vi "Create Grid.vi"(9 "Height":i32, 10 "Width":i32, 11 "Bounding Coordinates":T3={"Top Left Coordinate"={"Coordinate"=-3.0+1.5i, "Iteration"=0.0, "Escaped? "=FALSE, "Iteration Value"=0.0+0.0i}, "Bottom Right Coordinate"={"Coordinate"=1.0-1.5i, "Iteration"=0.0, "Escaped? "=FALSE, "Iteration Value"=0.0+0.0i}}) -> (3 "Grid":T1[][](array[typedef]))   [LabVIEW 2016]
uses:
  MandelPoint.ctl
panel:
  in  "MandelPointn Dummy":T1
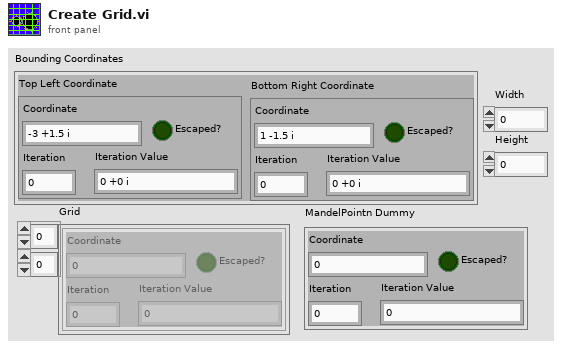
[diagram p1: front panel]
types:
  T1 = typedef "MandelPoint.ctl" = cluster{"Coordinate":cdb, "Iteration":u16, "Escaped? ":bool, "Iteration Value":cdb}
  T2 = typedef "MandelPoint.ctl" = cluster{"Coordinate":cdb, "Iteration":dbl, "Escaped? ":bool, "Iteration Value":cdb}
  T3 = cluster{"Top Left Coordinate":T2, "Bottom Right Coordinate":T2}
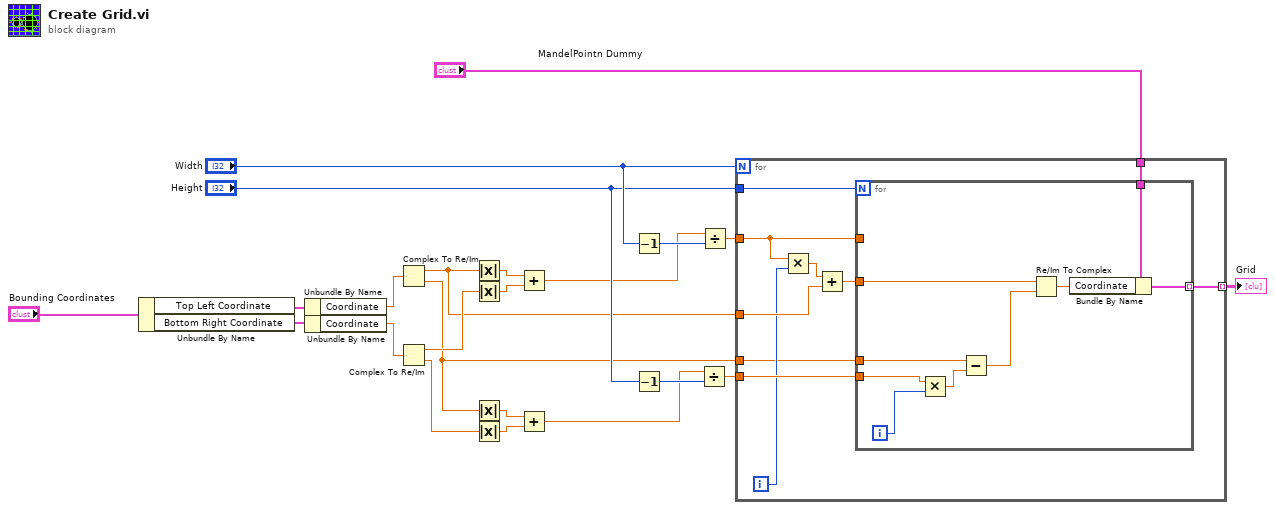
[diagram p0: block diagram]
diagram:
  n1 = Unbundle By Name("Bounding Coordinates") -> ("Top Left Coordinate"=w22:T2, "Bottom Right Coordinate"=w21:T2)
  n2 = Unbundle By Name(w22) -> ("Coordinate"=w16:cdb)
  n3 = Unbundle By Name(w21) -> ("Coordinate"=w15:cdb)
  n4 = Complex To Re/Im(x + iy=w16) -> (x=w3:dbl, y=w1:dbl)
  n5 = Complex To Re/Im(x + iy=w15) -> (x=w7:dbl, y=w2:dbl)
  n6 = Absolute Value(x=w3) -> (abs(x)=w10:dbl)
  n7 = Absolute Value(x=w7) -> (abs(x)=w9:dbl)
  n8 = Absolute Value(x=w1) -> (abs(x)=w6:dbl)
  n9 = Absolute Value(x=w2) -> (abs(x)=w5:dbl)
  n10 = Add(x=w10, y=w9) -> (x+y=w8:dbl)
  n11 = Add(x=w6, y=w5) -> (x+y=w4:dbl)
  n12 = Decrement(x="Width") -> (x-1=w13:i32)
  n13 = Decrement(x="Height") -> (x-1=w11:i32)
  n14 = Divide(x=w4, y=w11) -> (x/y=w19:dbl)
  n15 = Divide(x=w8, y=w13) -> (x/y=w20:dbl)
  n16 = for {
    N: "Width" -> [_]
    tunnel: "Height" -> [w33]
    tunnel: w3 -> [w31]
    tunnel: w1 -> [w26]
    tunnel: w20 -> [w29]
    tunnel: w19 -> [w32]
    tunnel: "MandelPointn Dummy" -> [w25]
    tunnel: [w24] -> w17 mode=indexing
    i -> [w28]
    n17 = Multiply(x=w29, y=w28) -> (x*y=w30:dbl)
    n18 = Add(x=w30, y=w31) -> (x+y=w27:dbl)
    n19 = for {
      N: w33 -> [_]
      tunnel: w29 -> [_]
      tunnel: w32 -> [w41]
      tunnel: w27 -> [w36]
      tunnel: w26 -> [w39]
      tunnel: w25 -> [w38]
      tunnel: [w34] -> w24 mode=indexing
      i -> [w40]
      n20 = Multiply(x=w41, y=w40) -> (x*y=w42:dbl)
      n21 = Subtract(x=w39, y=w42) -> (x-y=w35:dbl)
      n22 = Re/Im To Complex(1:w35, 2:w36) -> (0:w37:cdb)
      n23 = Bundle By Name(cluster=w38, "Coordinate"=w37) -> (w34:T1)
    }
  }
  "Grid" <- w17
